vi "PC Rio Data recieving test.vi"() -> ()   [LabVIEW 2017]
panel:
  out "PC To Rio":T1
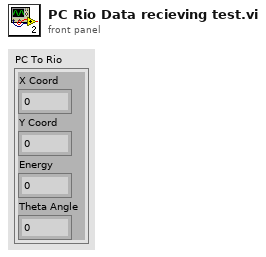
[diagram p1: front panel]
types:
  T1 = cluster{"X Coord":dbl, "Y Coord":dbl, "Energy":dbl, "Theta Angle":dbl}
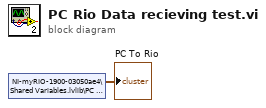
[diagram p0: block diagram]
diagram:
  n1 = shared-variable "NI-myRIO-1900-03050ae4\\Shared Variables.lvlib\\PC To Rio"() -> (→"PC To Rio":T1)  [unwired: 1 in, 1 out]
